vi "Terminate.vi"(8 "error in (no error)":errorcluster, 10 "Message in":refnum<class "TerminateMessage.lvclass">, 11 "Thorcam in":refnum<class "Thorcam.lvclass">) -> (0 "error out":errorcluster, 3 "Thorcam out":refnum<class "Thorcam.lvclass">)   [LabVIEW 2012, in "Thorcam.lvclass"]
doc: "This member function is called when the statemachine in the run.vi receives an 'terminate' command. It closes the RabbitMQ connection. \n\nOverride this member function in your derived class to release all previously acquired resources (but don't forget to call the parent method). If your component has subcomponents, they count as resources, and you have to release them by calling their own terminate functions."
uses:
  Thorcam.lvclass
  <vilib>/Distrio/Murmex/Murmex/Murmex.lvclass
  <vilib>/Distrio/Murmex/TerminateMessage/TerminateMessage.lvclass
panel:
  # "This method is called when the TERMINATE\ntrigger is sent. \n\nOverride this method when your component needs to\nrespond to this trigger. \n\nCall parent for proper implementation"
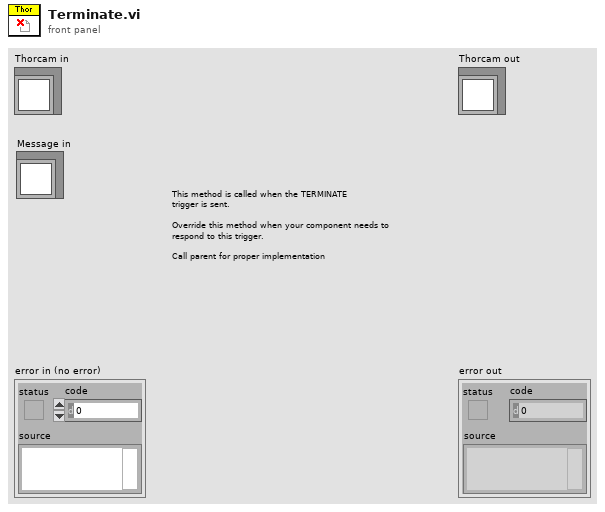
[diagram p1: front panel]
types:
  T1 = typedef "IMAQ Image.ctl" = refnum<image>
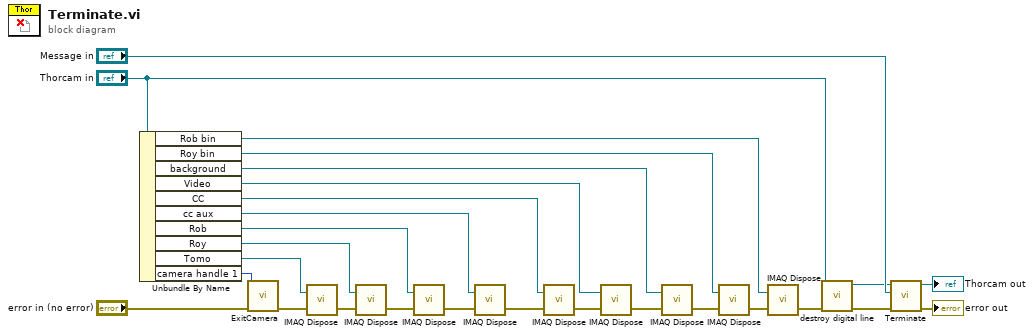
[diagram p0: block diagram]
diagram:
  n1 = Unbundle By Name("Thorcam in") -> ("Rob bin"=w5:T1, "Roy bin"=w6:T1, "background"=w9:T1, "Video"=w10:T1, "CC"=w11:T1, "cc aux"=w12:T1, "Rob"=w13:T1, "Roy"=w14:T1, "Tomo"=w15:T1, "camera handle 1"=w23:u32)
  n2 = call <instrlib>:"ExitCamera.vi"("error in"="error in (no error)", "Camera Handle In"=w23) -> ("error out"=w16:errorcluster)  [unwired: 9 in]
  n3 = call "IMAQ Dispose"("Image"=w15, "error in (no error)"=w16) -> ("error out"=w21:errorcluster)  [unwired: 4 in]
  n4 = call "IMAQ Dispose"("Image"=w14, "error in (no error)"=w21) -> ("error out"=w20:errorcluster)  [unwired: 4 in]
  n5 = call "IMAQ Dispose"("Image"=w13, "error in (no error)"=w20) -> ("error out"=w22:errorcluster)  [unwired: 4 in]
  n6 = call "IMAQ Dispose"("Image"=w12, "error in (no error)"=w22) -> ("error out"=w19:errorcluster)  [unwired: 4 in]
  n7 = call "IMAQ Dispose"("Image"=w11, "error in (no error)"=w19) -> ("error out"=w18:errorcluster)  [unwired: 4 in]
  n8 = call "IMAQ Dispose"("Image"=w10, "error in (no error)"=w18) -> ("error out"=w17:errorcluster)  [unwired: 4 in]
  n9 = call "IMAQ Dispose"("Image"=w9, "error in (no error)"=w17) -> ("error out"=w7:errorcluster)  [unwired: 4 in]
  n10 = call "IMAQ Dispose"("Image"=w6, "error in (no error)"=w7) -> ("error out"=w8:errorcluster)  [unwired: 4 in]
  n11 = call "IMAQ Dispose"("Image"=w5, "error in (no error)"=w8) -> ("error out"=w2:errorcluster)  [unwired: 4 in]
  n12 = call-dynamic "destroy digital line.vi"("error in (no error)"=w2, "Thorcam in"="Thorcam in") -> ("error out"=w1:errorcluster, "Thorcam out"=w3:refnum<class "Thorcam.lvclass">)  [unwired: 8 in]
  n13 = call-parent "Terminate.vi"("error in (no error)"=w1, "Message in"="Message in", "Murmex in"=w3) -> ("error out"=→"error out":errorcluster, "Murmex out"=→"Thorcam out":refnum<class "Thorcam.lvclass">)  [unwired: 7 in]
